vi "exp7foc7 (1).vi"() -> ()   [LabVIEW 2022 SP3]
uses:
  <vilib>/express/express arith-compare/Formula/XNode/ExpressFormulaBlockNode.xnode
panel:
  out "Boolean":bool
  out "System margin in ns":dbl(knob) scale=0.0..10.0
  out "Allowed system rise time delay in ns":dbl(knob) scale=0.0..10.0
  in  "Enum":enum16{"", "RZ", "NRZ"}(ring)
  in  "recevier bandwidth in GHZ":dbl(slide) scale=0.0..10.0
  in  "rise time in modal in ns":dbl(slide) scale=0.0..0.1
  in  "rise time of GVD":dbl(slide) scale=0.0..0.1
  in  "rise time of receving in ns":dbl(slide) scale=0.0..0.2
  in  "Rise time of transmitter in ns":dbl(slide) scale=0.0..0.1
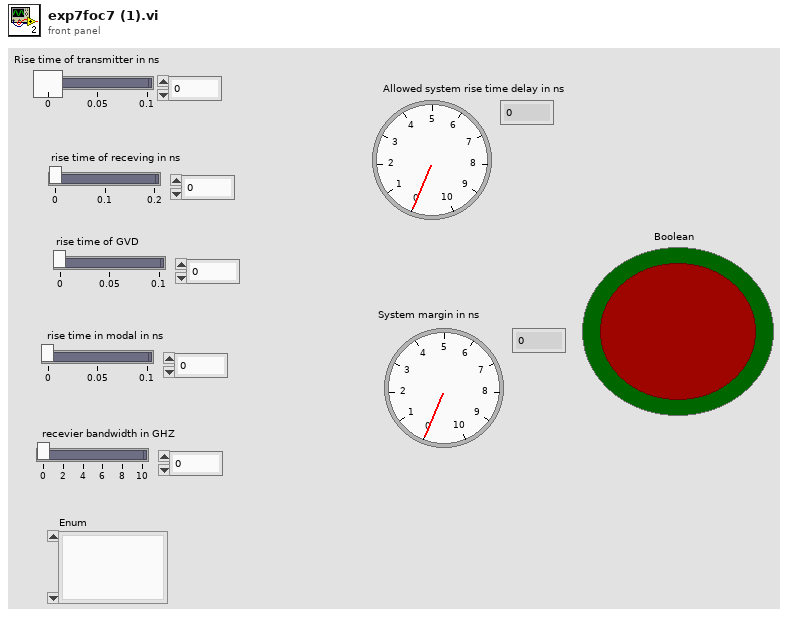
[diagram p1: front panel]
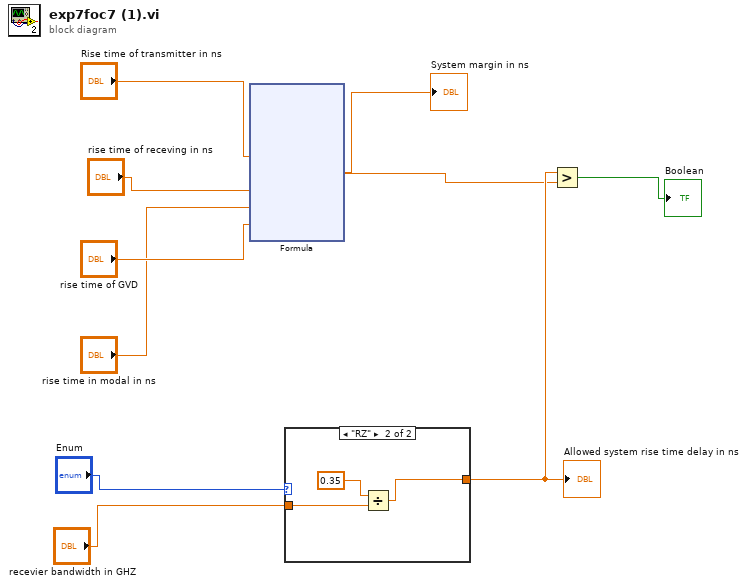
[diagram p0: block diagram]
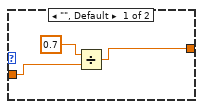
[diagram p2: hidden frame]
diagram:
  n1 = xnode "Formula"("Tt"="Rise time of transmitter in ns", "Tr"="rise time of receving in ns", "Tmodal"="rise time in modal in ns", "Tgvd"="rise time of GVD") -> ("Result"=w2:dbl)  [unwired: 1 in, 1 out]
  "System margin in ns" <- w2
  n2 = case shown="\"RZ\"" "Enum" {
    tunnel: "recevier bandwidth in GHZ" -> [w12 w14]
    tunnel: [w10 w13] -> w3
    frame "", Default {
      n3 = Divide(x=0.7 ("y"), y=w12) -> (x/y=w10:dbl)
    }
    frame "RZ" {
      n4 = Divide(x=0.35 ("y"), y=w14) -> (x/y=w13:dbl)
    }
  }
  "Allowed system rise time delay in ns" <- w3
  n5 = Greater?(x=w3, y=w2) -> (0:→"Boolean":bool)
